vi "Contour Line (Scalar).vi"(8 "height":dbl, 9 "Z":dbl[][](array[numeric]), 10 "Y":dbl[](array[numeric]), 11 "X":dbl[](array[numeric])) -> (0 "error":i32, 2 "Contour Line":T1, 3 "Contour Graph":cluster{dbl[], dbl[]}(graph))   [LabVIEW 2020, in "NI_AAL_Geometry.lvlib"]
doc: "Calculates and returns the contour lines of a surface and the contour graph."
uses:
  <vilib>/Analysis/NI_AAL_Geometry.lvlib
  <vilib>/Analysis/geometry.llb/Contour Lines Control.ctl
  <vilib>/Analysis/geometry.llb/Contour Line Segment.ctl
  <vilib>/gmath/interp.llb/Create Mesh Grid (2D) (x,y arrays).vi
  <vilib>/gmath/NI_Gmath.lvlib
panel:
  # "Contour Line"
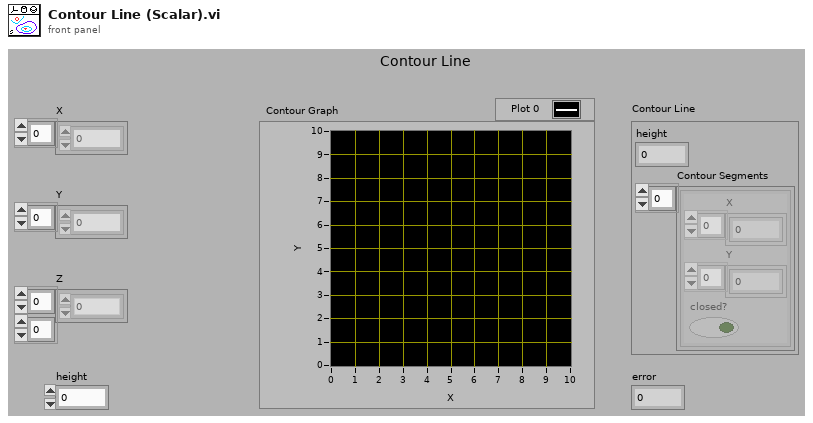
[diagram p1: front panel]
types:
  T1 = typedef "NI_AAL_Geometry.lvlib/Contour Lines Control.ctl" = cluster{"height":dbl, "Contour Segments":T2[]}
  T2 = typedef "NI_AAL_Geometry.lvlib/Contour Line Segment.ctl" = cluster{"X":dbl[], "Y":dbl[], "closed?":bool}
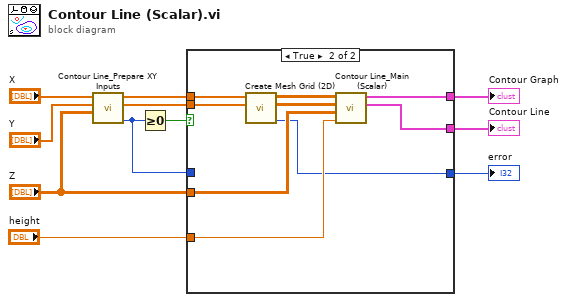
[diagram p0: block diagram]
diagram:
  n1 = call <vilib>:"Contour Line_Prepare XY Inputs.vi"("Z In"="Z", "Y In"="Y", "X In"="X") -> ("error"=w2:i32, "Y Out"=w4:dbl[], "X Out"=w5:dbl[])  [unwired: 6 in]
  n2 = Greater Or Equal To 0?(x=w2) -> (x >= 0?=w3:bool)
  n3 = case shown="True" w3 {
    tunnel: "height" -> [_ w16]
    tunnel: [_ w15] -> w10
    tunnel: w5 -> [_ w21]
    tunnel: "Z" -> [_ w17]
    tunnel: [_ w14] -> w9
    tunnel: w4 -> [_ w20]
    tunnel: [w12 w13] -> w1
    tunnel: w2 -> [w12 _]
    frame False {
    }
    frame True {
      n4 = call-poly <vilib>:"Create Mesh Grid (2D).vi"("y domain"=w20, "x domain"=w21) -> ("error"=w13:i32, "Y"=w18:dbl[][], "X"=w19:dbl[][])  [unwired: 7 in]
      n5 = call <vilib>:"Contour Line_Main (Scalar).vi"("height"=w16, "Z"=w17, "Y"=w18, "X"=w19) -> ("Contour Line"=w14:T1, "Contour Graph"=w15:cluster{dbl[], dbl[]})  [unwired: 6 in]
    }
  }
  "error" <- w1
  "Contour Graph" <- w10
  "Contour Line" <- w9
